vi "Pre Launch Init.vi"(11 "Measurement in":refnum<class "Measurement.lvclass">) -> (0 "error out":errorcluster, 3 "Measurement out":refnum<class "Measurement.lvclass">)   [LabVIEW 2020, in "Measurement.lvlib" / "Measurement.lvclass"]
doc: "(<B>Filename</B>: Actor Framework.lvlib:Actor.lvclass:Pre Launch Init.vi)\n\nDefines behavior that occurs after the Launch Nested Actor method is invoked but before the actor's Actor Core method begins running.\n\nBy default, this method does nothing. A descendant class may override it to define behavior."
uses:
  Measurement.lvclass
  Measurement.lvclass/Measurement.ctl
  <vilib>/ActorFramework/Actor/Actor.lvclass
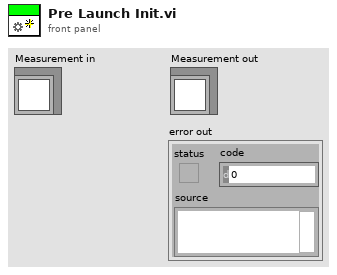
[diagram p1: front panel]
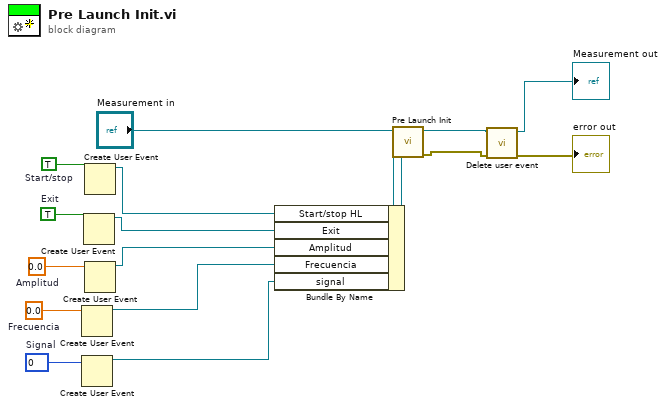
[diagram p0: block diagram]
diagram:
  w8 = u16 0 items=[""]  # Signal
  w9 = 0.0  # Frecuencia
  w10 = 0.0  # Amplitud
  w12 = TRUE  # Exit
  w14 = TRUE  # Start/stop
  n1 = Create User Event(user event datatype=w9) -> (user event=w6:refnum<user-event>)  [unwired: 1 in, 1 out]
  n2 = Create User Event(user event datatype=w8) -> (user event=w5:refnum<user-event>)  [unwired: 1 in, 1 out]
  n3 = Create User Event(user event datatype=w12) -> (user event=w11:refnum<user-event>)  [unwired: 1 in, 1 out]
  n4 = Create User Event(user event datatype=w14) -> (user event=w13:refnum<user-event>)  [unwired: 1 in, 1 out]
  n5 = Create User Event(user event datatype=w10) -> (user event=w7:refnum<user-event>)  [unwired: 1 in, 1 out]
  n6 = Bundle By Name(cluster="Measurement in", "Start/stop HL"=w13, "Exit"=w11, "Amplitud"=w7, "Frecuencia"=w6, "signal"=w5) -> (w15:refnum<class "Measurement.lvclass">)
  n7 = call-parent "Pre Launch Init.vi"("Actor in"=w15) -> ("error out"=w4:errorcluster, "Actor out"=w2:refnum<class "Measurement.lvclass">)  [unwired: 9 in]
  n8 = call "Delete user event.vi"("error in (no error)"=w4, "Measurement in"=w2) -> ("error out"=→"error out":errorcluster, "Measurement out"=→"Measurement out":refnum<class "Measurement.lvclass">)  [unwired: 8 in]
